vi "MT Open Net.vi"(6 "IPPort":u16, 7 "IP3":u8, 9 "IP2":u8, 10 "IP1":u8, 11 "IP0":u8) -> (3 "function return":i32)   [LabVIEW 2014, in "MT_API.lvlib"]
doc: "MT_API INT32 __stdcall MT_Open_Net(BYTE IP0,BYTE IP1,BYTE IP2,BYTE IP3,WORD IPPort);"
uses:
  MT_API.lvlib
  MT_API.dll
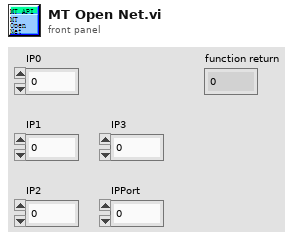
[diagram p1: front panel]
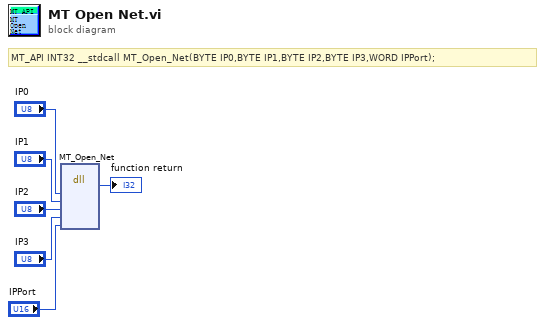
[diagram p0: block diagram]
diagram:
  # "MT_API INT32 __stdcall MT_Open_Net(BYTE IP0,BYTE IP1,BYTE IP2,BYTE IP3,WORD IPPort);"
  n1 = dll-call lib="E:/Projects/LabView/MT_API/MT_API.*" fn="MT_Open_Net"("IP0"="IP0", "IP1"="IP1", "IP2"="IP2", "IP3"="IP3", "IPPort"="IPPort") -> (→"function return":i32)  [unwired: 8 in, 2 out]
